vi "test Get CPU Channels.vi"(8 "error in (no error)":errorcluster, 11 "TestCase in":refnum<class "System Monitor System Tests.lvclass">) -> (0 "error out":errorcluster, 3 "TestCase out":refnum<class "System Monitor System Tests.lvclass">)   [LabVIEW 2027, in "System Monitor System Tests.lvclass"]
uses:
  System Monitor System Tests.lvclass
  C:/Program Files/National Instruments/LabVIEW 2027/vi.lib/addons/_JKI Toolkits/VI Tester/TestCase.llb/TestCase.lvclass
  <vilib>/addons/_JKI Toolkits/VI Tester/TestCase.llb/TestCase.lvclass
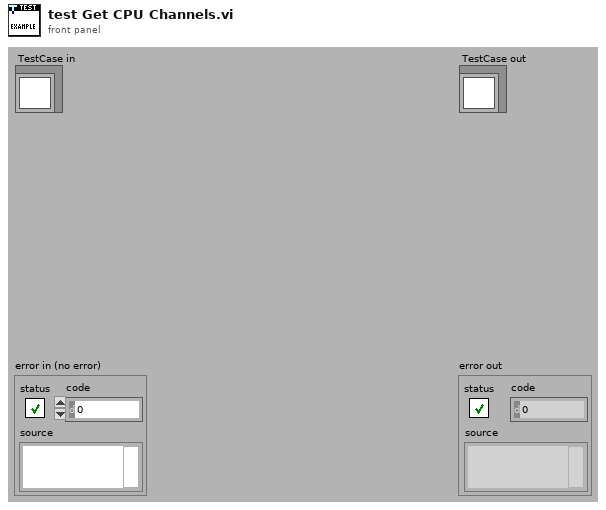
[diagram p1: front panel]
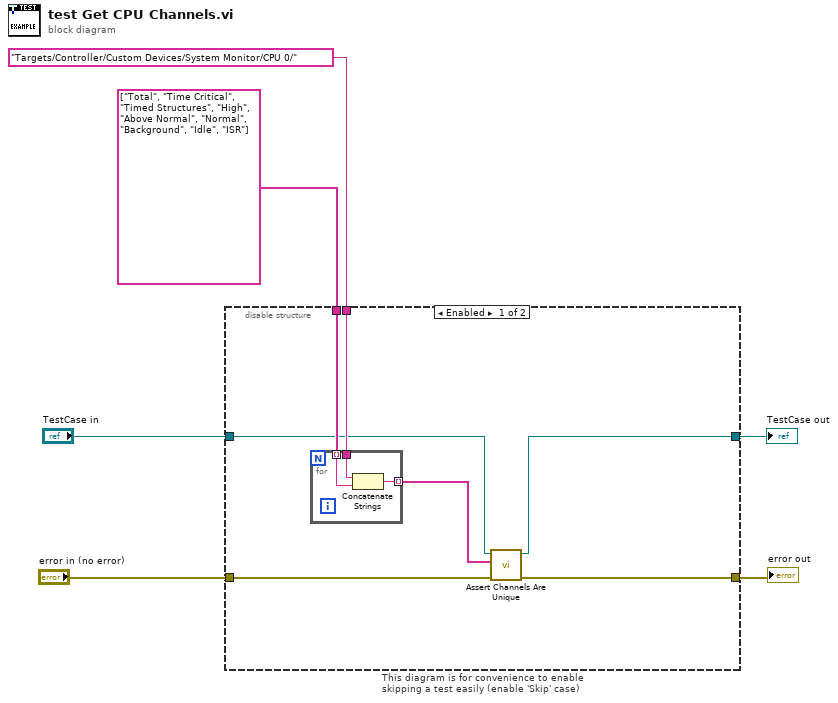
[diagram p0: block diagram]
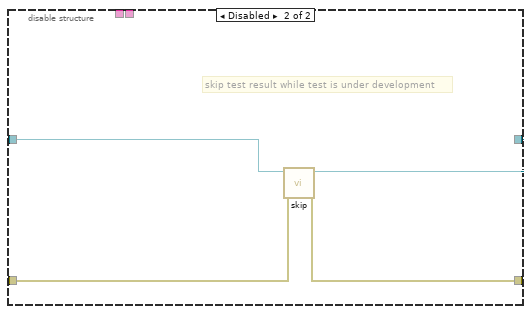
[diagram p2: hidden frame]
diagram:
  n1 = disable-structure "This diagram is for convenience to enable skipping a test easily (enable 'Skip' case)" shown="Enabled" {
    disable-tunnel: "TestCase in" -> [w9 w20]
    disable-tunnel: [w8 w18] -> w3
    disable-tunnel: [w7 w19] -> w5
    disable-tunnel: "error in (no error)" -> [w11 w17]
    disable-tunnel: string[] ["Total", "Time Critical", "Timed Structures", "High", "Above Normal", "Normal", "Background", "Idle", "ISR"] -> [w13 _]
    disable-tunnel: "Targets/Controller/Custom Devices/System Monitor/CPU 0/" ("Channel") -> [w12 _]
    frame Enabled {
      n2 = for {
        tunnel: w13 -> [w16] mode=indexing
        tunnel: [w15] -> w10 mode=indexing
        tunnel: w12 -> [w14]
        n3 = Concatenate Strings(w14, w16) -> (w15:string)
      }
      n4 = call "Assert Channels Are Unique.vi"("error in (no error)"=w11, "Channels in"=w10, "System Monitor System Tests in"=w9) -> ("error out"=w7:errorcluster, "System Monitor System Tests out"=w8:refnum<class "System Monitor System Tests.lvclass">)  [unwired: 7 in]
    }
    frame Disabled {
      # "skip test result while test is under development"
      n5 = call <vilib>:"skip.vi"("error in (no error)"=w17, "TestCase in"=w20) -> ("error out"=w19:errorcluster, "TestCase out"=w18:refnum<class "System Monitor System Tests.lvclass">)  [unwired: 8 in]
    }
  }
  "error out" <- w5
  "TestCase out" <- w3
